vi "Fetch List Items From Table (SubVI).vi"(3 "error IN":errorcluster, 4 "ColumnName":string=" ", 5 "TableName":string) -> (0 "error OUT":errorcluster, 2 "recordset data":string[][](array[string]))   [LabVIEW 2010]
uses:
  <vilib>/addons/database/Connection.llb/DB Tools Open Connec (Path).vi
  <vilib>/addons/database/Connection.llb/Conn Execute.vi
  <vilib>/addons/database/Recordset.llb/Rec Destroy - Connection.vi
  <vilib>/addons/database/NI_Database_API.lvlib
panel:
  out "SP Call":string
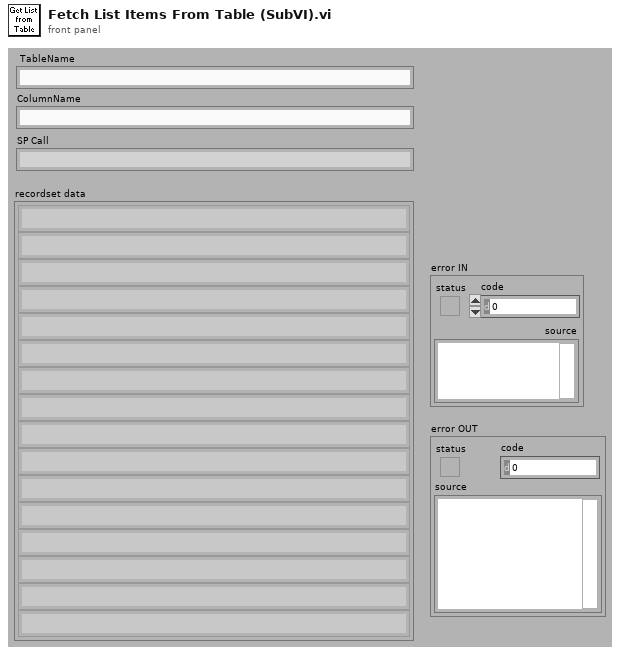
[diagram p1: front panel]
types:
  T1 = typedef "NI_Database_API.lvlib/Conn ObjectReference.ctl" = refnum<k1>
  T2 = typedef "NI_Database_API.lvlib/Rec ObjectReference.ctl" = refnum<k1>
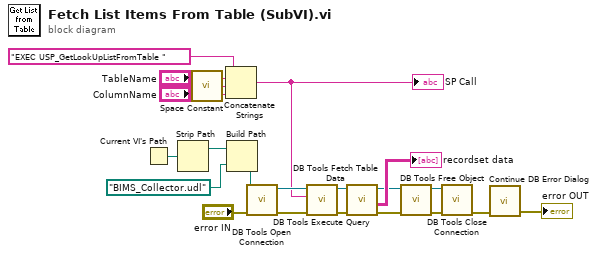
[diagram p0: block diagram]
diagram:
  n1 = Current VI's Path() -> (path=w9:path)
  n2 = Strip Path(path=w9) -> (stripped path=w8:path)  [unwired: 1 out]
  n3 = call <vilib>:"Space Constant.vi"() -> ("String"=w1:string)
  n4 = Concatenate Strings("EXEC USP_GetLookUpListFromTable " ("string"), "TableName", w1, "ColumnName") -> (w4:string)
  "SP Call" <- w4
  n5 = Build Path(base path=w8, name or relative path=path "BIMS_Collector.udl" ("connectString")) -> (appended path=w6:path)
  n6 = call-poly <vilib>:"DB Tools Open Connection.vi"("error in (no error)"="error IN", "connection information"=w6) -> ("error out"=w14:errorcluster, "connection reference"=w12:T1)  [unwired: 6 in]
  n7 = call-poly <vilib>:"DB Tools Execute Query.vi"("error in (no error)"=w14, "SQL query"=w4, "connection reference"=w12) -> ("error out"=w15:errorcluster, "recordset reference"=w11:T2)  [unwired: 5 in]
  n8 = call <vilib>:"DB Tools Fetch Table Data.vi"("error in (no error)"=w15, "recordset reference"=w11) -> ("error out"=w16:errorcluster, "recordset data"=→"recordset data":string[][], "recordset reference out"=w10:T2)  [unwired: 3 in]
  n9 = call-poly <vilib>:"DB Tools Free Object.vi"("error in (no error)"=w16, "recordset reference"=w10) -> ("error out"=w17:errorcluster, "connection reference"=w13:T1)  [unwired: 8 in]
  n10 = call <vilib>:"DB Tools Close Connection.vi"("error in (no error)"=w17, "connection reference"=w13) -> ("error out"=w19:errorcluster)  [unwired: 5 in]
  n11 = call "Continue DB Error Dialog.vi"("error in (no error)"=w19) -> ("error out"=→"error OUT":errorcluster)  [unwired: 3 in, 2 out]
